vi "UTF8_ASCI.vi"(8 "error in (no error)":errorcluster, 11 "Array":string[][](array[string])) -> (0 "error out":errorcluster, 3 "Array 2":string[][](array[string]))   [LabVIEW 2018, in "Controller.lvlib"]
uses:
  Controller.lvlib
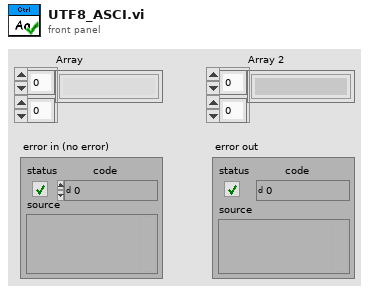
[diagram p1: front panel]
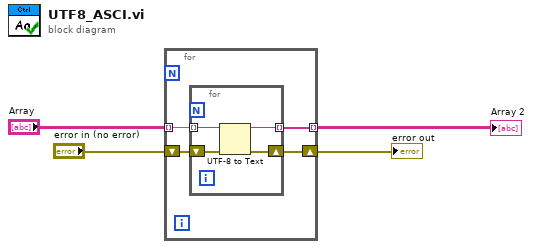
[diagram p0: block diagram]
diagram:
  n1 = for {
    tunnel: "Array" -> [w8] mode=indexing
    tunnel: [w7] -> w3 mode=indexing
    shift-right: [w5] -> w1
    shift-left: "error in (no error)" -> [w6]
    n2 = for {
      tunnel: w8 -> [w12] mode=indexing
      tunnel: [w11] -> w7 mode=indexing
      shift-right: [w9] -> w5
      shift-left: w6 -> [w10]
      n3 = UTF-8 to Text(8:w10, 11:w12) -> (0:w9:errorcluster, 3:w11:string)  [unwired: 1 in]
    }
  }
  "Array 2" <- w3
  "error out" <- w1
